vi "CC Script Parse Dither.vi"(8 "error in (no error)":errorcluster, 9 "To String?":bool, 10 "Dithering in":T1={"Name"="", "Dithering Offsets"={"Offsets"=[{"DEC"=0.0, "RA"=0.0}, {"DEC"=-10.0, "RA"=-10.0}]}}, 11 "Dither Parameters":string="\"Rnadome Dither Mispeller\" Count=3,Radius=1.23") -> (0 "error out":errorcluster, 2 "Dithering out":T1, 3 "resulting string":string)   [LabVIEW 2024]
uses:
  typedefs/CC Dithering.ctl
  typedefs/CC cluster Offset Dithering.ctl
  typedefs/CC Dithering Offsets.ctl
  typedefs/CC enum Dithering Types.ctl
  <vilib>/regexp/Match Regular Expression.xnode
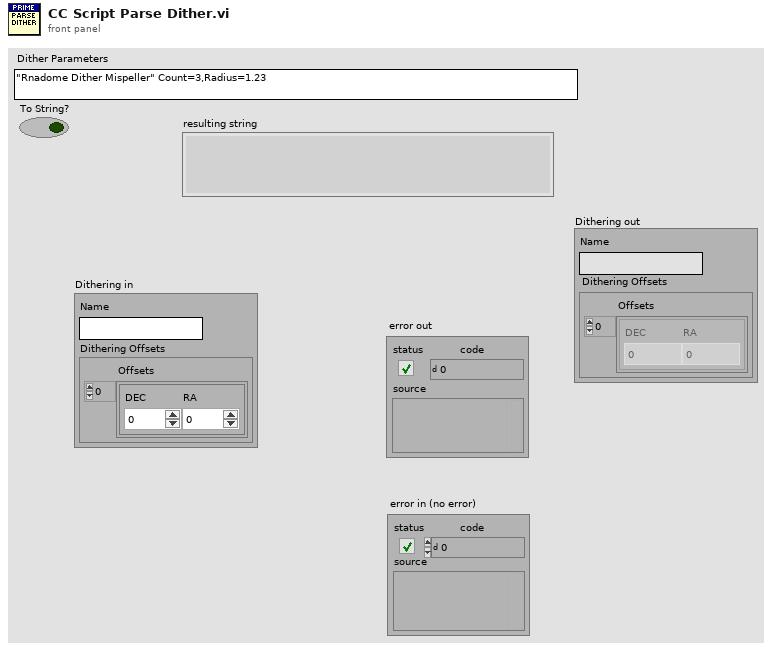
[diagram p1: front panel]
types:
  T1 = typedef "CC Dithering.ctl" = cluster{"Name":string, "Dithering Offsets":T2}
  T2 = typedef "CC cluster Offset Dithering.ctl" = cluster{"Offsets":T3[]}
  T3 = typedef "CC Dithering Offsets.ctl" = cluster{"DEC":dbl, "RA":dbl}
  T4 = typedef "CC enum Dithering Types.ctl" = enum16{"Random", "Offsets", "None"}
  T5 = typedef "CC cluster Random Dithering.ctl" = cluster{"Count":i32, "Radius":dbl, "Name":string}
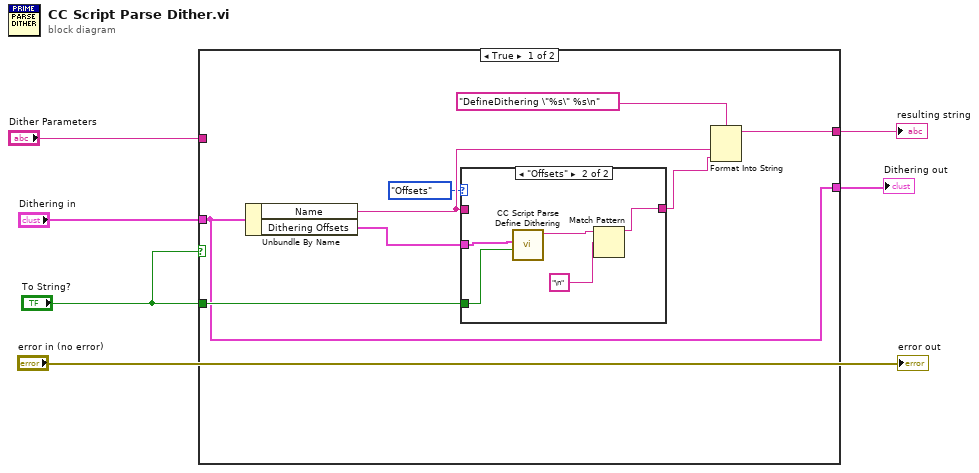
[diagram p0: block diagram]
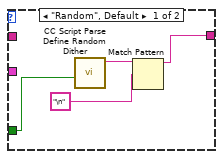
[diagram p2: hidden frame]
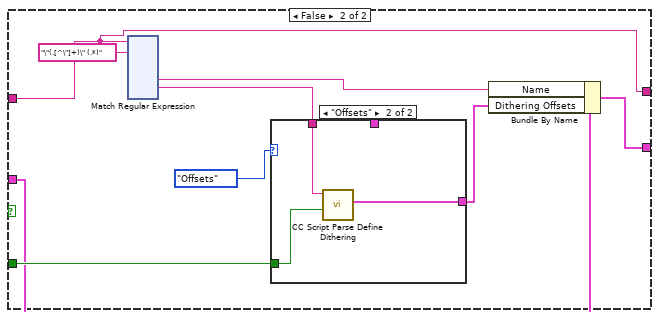
[diagram p3: hidden frame]
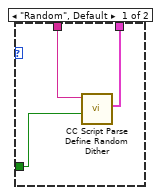
[diagram p4: hidden frame]
diagram:
  n1 = case shown="True" "To String?" {
    tunnel: "Dithering in" -> [w10 w30]
    tunnel: [w14 w27] -> w4
    tunnel: "Dither Parameters" -> [_ w27]
    tunnel: "To String?" -> [w13 w32]
    tunnel: [w10 w28] -> w1
    frame True {
      n2 = Unbundle By Name(w10) -> ("Name"=w8:string, "Dithering Offsets"=w12:T2)
      n3 = case shown="\"Offsets\"" CC_enum_Dithering_Types."Offsets" ("Dithering Type") {
        tunnel: w12 -> [_ w23]
        tunnel: [w15 w19] -> w11
        tunnel: w8 -> [_ _]
        tunnel: w13 -> [w16 w20]
        frame "Random", Default {
          n4 = call "CC Script Parse Define Random Dither.vi"("To String?"=w16) -> ("Script String out"=w17:string)  [unwired: 8 in, 2 out]
          n5 = Match Pattern(string=w17, regular expression="\n") -> (before substring=w15:string)  [unwired: 1 in, 3 out]
        }
        frame "Offsets" {
          n6 = call "CC Script Parse Define Dithering.vi"("To Script?"=w20, "Dithering Offsets in"=w23) -> ("Script out"=w21:string)  [unwired: 7 in, 2 out]
          n7 = Match Pattern(string=w21, regular expression="\n") -> (before substring=w19:string)  [unwired: 1 in, 3 out]
        }
      }
      n8 = Format Into String(format string="DefineDithering \"%s\" %s\n", w8, w11) -> (resulting string=w14:string)  [unwired: 2 in, 1 out]
    }
    frame False {
      n9 = xnode "Match Regular Expression"("input string"=w27, "regular expression"="\"(.[^\"]+)\" (.*)") -> ("submatch 1"=w25:string, "submatch 2"=w24:string)  [unwired: 4 in, 6 out]
      n10 = case shown="\"Offsets\"" CC_enum_Dithering_Types."Offsets" ("output 1") {
        tunnel: w32 -> [w156 w159]
        tunnel: w24 -> [w154 w158]
        tunnel: [_ w157] -> w29
        tunnel: [w155 _] -> _
        frame "Random", Default {
          n11 = call "CC Script Parse Define Random Dither.vi"("To String?"=w156, "Dither Parameters"=w154) -> ("Random Dither out"=w155:T5)  [unwired: 7 in, 2 out]
        }
        frame "Offsets" {
          n12 = call "CC Script Parse Define Dithering.vi"("To Script?"=w159, "DefineDithering Parameters"=w158) -> ("Dithering Offsets out"=w157:T2)  [unwired: 7 in, 2 out]
        }
      }
      n13 = Bundle By Name(cluster=w30, "Name"=w25, "Dithering Offsets"=w29) -> (w28:T1)
    }
  }
  "resulting string" <- w4
  "Dithering out" <- w1
  "error out" <- "error in (no error)"
